vi "CompressorEnabled.vi"() -> ()   [LabVIEW 2019]
uses:
  <vilib>/Rock Robotics/WPI/Framework/Command Status Info.ctl
  <vilib>/Rock Robotics/WPI/Framework/Completion Status.ctl
  <vilib>/Rock Robotics/WPI/Framework/Completion Notifier.ctl
  Implementation/Pnuematics Setpoints.ctl
  Implementation/Pnuematics Operations.ctl
  <vilib>/Rock Robotics/WPI/Solenoid/WPI_SolenoidValue.ctl
panel:
  in  "Description":string="Reserve"
  in  "Command Name":string
  out "Command Info":T1
  in  "Command Info 2":T1
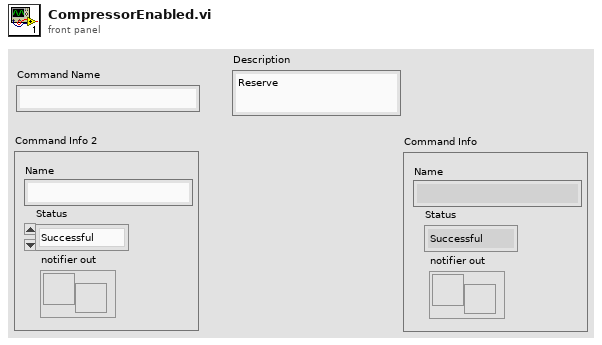
[diagram p1: front panel]
types:
  T1 = typedef "Command Status Info.ctl" = cluster{"Name":string, "Status":T2, "notifier out":T3}
  T2 = typedef "Completion Status.ctl" = enum16{"Successful", "Aborted", "Incomplete"}
  T3 = typedef "Completion Notifier.ctl" = refnum<notifier>
  T4 = typedef "Pnuematics Setpoints.ctl" = cluster{"Operation":T5, "Value":T6, "Solenoid":enum16{"Default", "Transmission", "Wheel"}, "Milliseconds":dbl}
  T5 = typedef "Pnuematics Operations.ctl" = enum16{"Reserve", "Read Current", "CompressorStart", "CompressorEnabled", "CompressorStop", "Solenoid", "Immediate"}
  T6 = typedef "WPI_SolenoidValue.ctl" = enum16{"Off", "On", "Forward", "Reverse"}
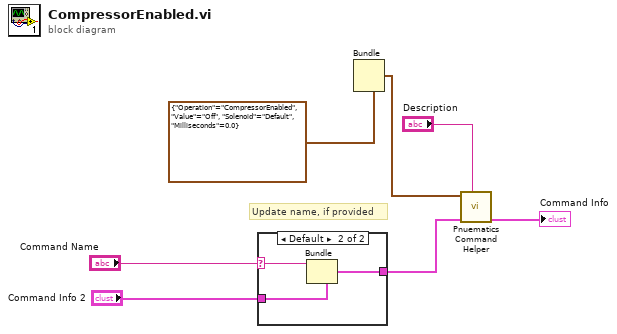
[diagram p0: block diagram]
diagram:
  # "Update name, if provided"
  n1 = case shown="Default" "Command Name" {
    selector: "Command Name" -> [_ w9]
    tunnel: "Command Info 2" -> [w8 w11]
    tunnel: [w8 w10] -> w4
    frame "" {
    }
    frame Default {
      n2 = Bundle(cluster=w11, "Name"=w9) -> (w10:T1)  [unwired: 2 in]
    }
  }
  n3 = Bundle(cluster=T4 {"Operation"=enum."CompressorEnabled", "Value"=enum."Off", "Solenoid"=enum."Default", "Milliseconds"=0.0} ("SubSystem Data")) -> (w1:T4)  [unwired: 4 in]
  n4 = call "Pnuematics Command Helper.vi"("Description"="Description", "Command Info In"=w4, "SubSystem Data"=w1) -> ("Command Info Out"=→"Command Info":T1)  [unwired: 6 in, 2 out]
